vi "set center freq.vi"(8 "error in (no error)":errorcluster, 10 "freq":u32, 11 "DevRefnum":u64) -> (0 "error out":errorcluster, 2 "freq":u32, 3 "DevRefnum":u64)   [LabVIEW 2013, in "rtlsdr.lvlib"]
doc: "RTLSDR_API int rtlsdr_set_center_freq(rtlsdr_dev_t *dev, uint32_t freq);"
uses:
  <instrlib>/rtlsdr/rtlsdr.lvlib
  <instrlib>/rtlsdr/VIs/rtlsdr.dll
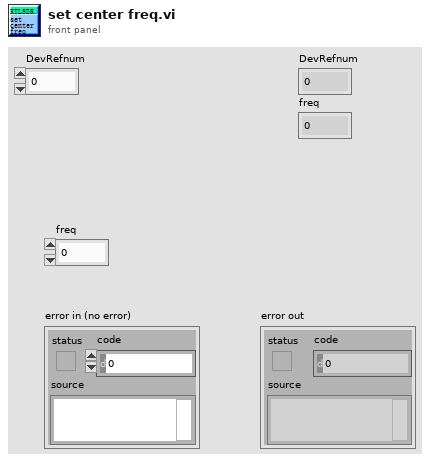
[diagram p1: front panel]
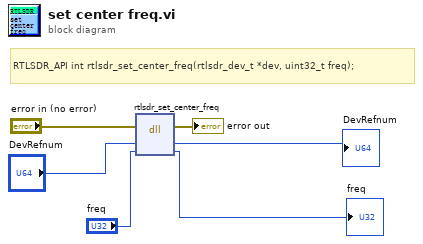
[diagram p0: block diagram]
diagram:
  # "RTLSDR_API int rtlsdr_set_center_freq(rtlsdr_dev_t *dev, uint32_t freq);"
  n1 = dll-call lib="C:/Program Files (x86)/National Instruments/LabVIEW 2013/instr.lib/rtlsdr/VIs/rtlsdr.*" fn="rtlsdr_set_center_freq"(error in="error in (no error)", "DevRefnum"="DevRefnum", "freq"="freq") -> (error out=→"error out":errorcluster, "DevRefnum"=→"DevRefnum":u64, "freq"=→"freq":u32)  [unwired: 3 in, 1 out]
